vi "pause after every move (global variable).vi"() -> ()   [LabVIEW 2020, in "core.lvlib"]
uses:
  core.lvlib
panel:
  out "pause core after every move?":bool
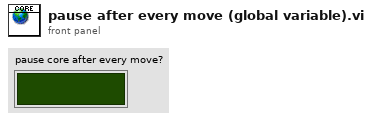
[diagram p1: front panel]
diagram:
